vi "ShareBus.vi"(9 "i1":fxp<+/-,25,5>, 10 "i2":fxp<+/-,25,5>, 11 "i3":fxp<+/-,25,5>) -> (3 "Vb":fxp<+,27,7>)   [LabVIEW 2015]
uses:
  <vilib>/rvi/FXPMathLib/FxpMul/XNode/nifxpmath_Multiplier.xnode
  <vilib>/rvi/FXPMathLib/sim/FxpSim.dll
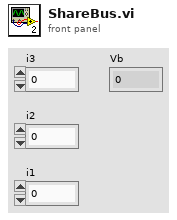
[diagram p1: front panel]
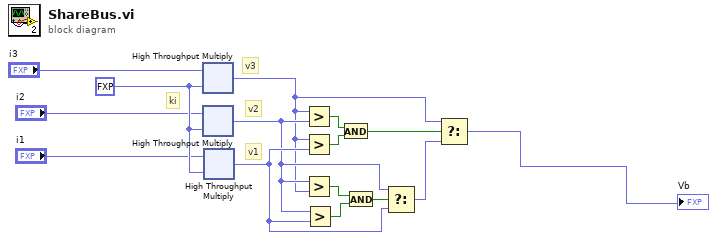
[diagram p0: block diagram]
diagram:
  w15 = fxp<+,3,3> 6.0 ("y")
  # "v1"
  # "v2"
  # "v3"
  # "ki"
  n1 = xnode "High Throughput Multiply"("x"="i3", "y"=w15) -> ("x*y"=w10:fxp<+,27,7>)
  n2 = xnode "High Throughput Multiply"("x"="i2", "y"=w15) -> ("x*y"=w12:fxp<+,27,7>)
  n3 = xnode "High Throughput Multiply"("x"="i1", "y"=w15) -> ("x*y"=w14:fxp<+,27,7>)
  n4 = Greater?(x=w10, y=w12) -> (0:w4:bool)
  n5 = Greater?(x=w10, y=w14) -> (0:w3:bool)
  n6 = Greater?(x=w12, y=w10) -> (0:w5:bool)
  n7 = Greater?(x=w12, y=w14) -> (0:w6:bool)
  n8 = And(x=w4, y=w3) -> (x .and. y?=w2:bool)
  n9 = And(x=w5, y=w6) -> (x .and. y?=w7:bool)
  n10 = Select(t=w12, s=w7, f=w14) -> (s? t:f=w8:fxp<+,27,7>)
  n11 = Select(t=w10, s=w2, f=w8) -> (s? t:f=→"Vb":fxp<+,27,7>)
